vi "get hallsensor settings.vi"(8 "error in (no error)":errorcluster, 10 "hallsensor_settings":T1, 11 "id":i32) -> (0 "error out":errorcluster, 2 "hallsensor_settings out":T1, 3 "function return":i32)   [LabVIEW 2012, in "libximc.lvlib"]
doc: "result_t XIMC_API get_hallsensor_settings (device_t id, hallsensor_settings_t* hallsensor_settings);"
uses:
  libximc.lvlib
  libximc.dll
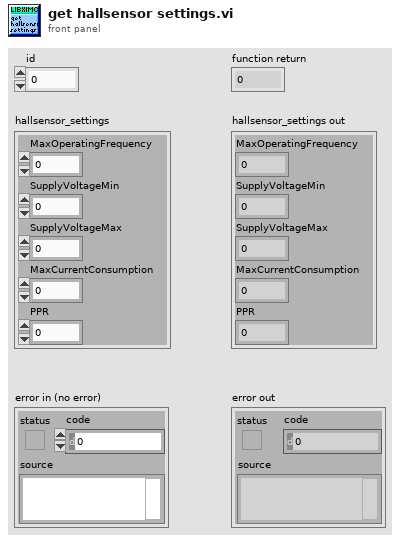
[diagram p1: front panel]
types:
  T1 = cluster{"MaxOperatingFrequency":sgl, "SupplyVoltageMin":sgl, "SupplyVoltageMax":sgl, "MaxCurrentConsumption":sgl, "PPR":u32}
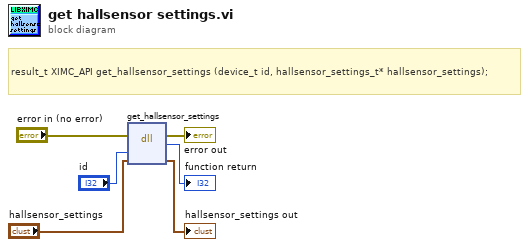
[diagram p0: block diagram]
diagram:
  # "result_t XIMC_API get_hallsensor_settings (device_t id, hallsensor_settings_t* hallsensor_settings);"
  n1 = dll-call lib="C:/Users/Stepan/Downloads/labview_2.9.11_testgen_thread/libximc.*" fn="get_hallsensor_settings"(error in="error in (no error)", "id"="id", "hallsensor_settings"="hallsensor_settings") -> (error out=→"error out":errorcluster, →"function return":i32, "hallsensor_settings"=→"hallsensor_settings out":T1)  [unwired: 3 in, 1 out]
